vi "CRYOperator Process.vi"(9 "VI ID":i32=-1, 10 "sAction":string, 11 "sOperator Type":string) -> (3 "Data String":string)   [LabVIEW 2013]
uses:
  Control/CRYOperator Configure Cluster.ctl
  <vilib>/Utility/miscctls.llb/LVRectTypeDef.ctl
  SubVI/CRYMisc vis settings global.vi
panel:
  in  "Operator All Cluster":T1
  # "Register Operator Window."
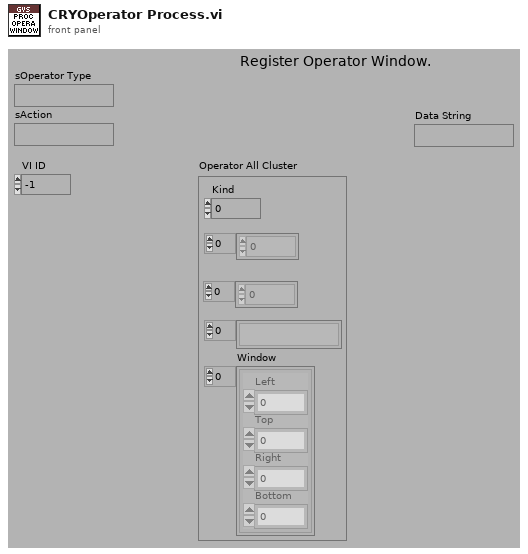
[diagram p1: front panel]
types:
  T1 = typedef "CRYOperator Configure Cluster.ctl" = cluster{"Kind":i32, "VI nID":i32[], "Title nID":i32[], "Setting":string[], "Window":T2[]}
  T2 = typedef "LVRectTypeDef.ctl" = cluster{"Left":i16, "Top":i16, "Right":i16, "Bottom":i16}
  T3 = cluster{"interactive":bool, "displayed":bool, "in a seq":bool}
  T4 = enum32{"Invalid", "Standard", "Closed", "Hidden", "Minimized", "Maximized"}
  T5 = enum32{"Invalid", "Default", "Floating", "Floating/Auto-Hide", "Modal"}
  T6 = cluster{"VI Ref":refnum<vi>[], "VI nID":i32[], "Title nID":i32[]}
  T7 = cluster{"gen'r mode":i32, "frequency":u32, "output level":dbl, "wave path":string, "wav play mode":i32, "duration":dbl, "n times":i32, "channel":i32, "wav level":dbl, "EQ":bool, "f knob log":bool, "f knob low":dbl, "f knob high":dbl, "ol knob log":bool, "ol knob low":dbl, "ol knob high":dbl, "Lin Display Prefs":string, "dB Display Prefs":string, "Duration noise":dbl, "Min freq noise":dbl, "Max freq noise":dbl, "Channel String":string, "Play Sine Wave":i32}
  T8 = typedef "CRYMultimeter.ctl" = cluster{"Ave/Max/Min":i32, "Level":i32, "Channel":i32, "Signal Type":string, "Weighting":string, "Applay Correction":bool, "lin/exp avg":u16, "rec time (sec)":dbl, "Average Time (Sec)":dbl, "Lin Display Prefs":string, "dB Display Prefs":string, "Time Weighting":u16, "Display":u16}
  T9 = typedef "CRYScope-FFT.ctl" = cluster{"window":i32, "n avgs":i32, "lin/exp avg":i32, "pwr/cplx avg":i32, "time (ms)":dbl, "fft lines":i32, "scope/fft mode":i32, "channel":i32, "trig. channel":i32, "Applay Correction":bool, "Time Display":string, "Freq. Weighting":string, "Ave/Max/Min":u16, "Trigger Level":dbl, "Trigger Unit":u16, "Trigger Time Offset":dbl, "Trigger Slope":u16, "Trigger/Free Run":bool, "continuous":bool, "Spectrum Display":string, "Calc FFT":bool, "Y-axis":string, "Signal Type":string}
  T10 = cluster{"octave":i32, "det time":i32, "det sec":dbl, "lin/exp":i32, "weighting":i32, "channel":i32, "Ave/Max/Min":u16, "continuous":bool, "Applay Correction":bool, "Display":u16, "Channel String":string}
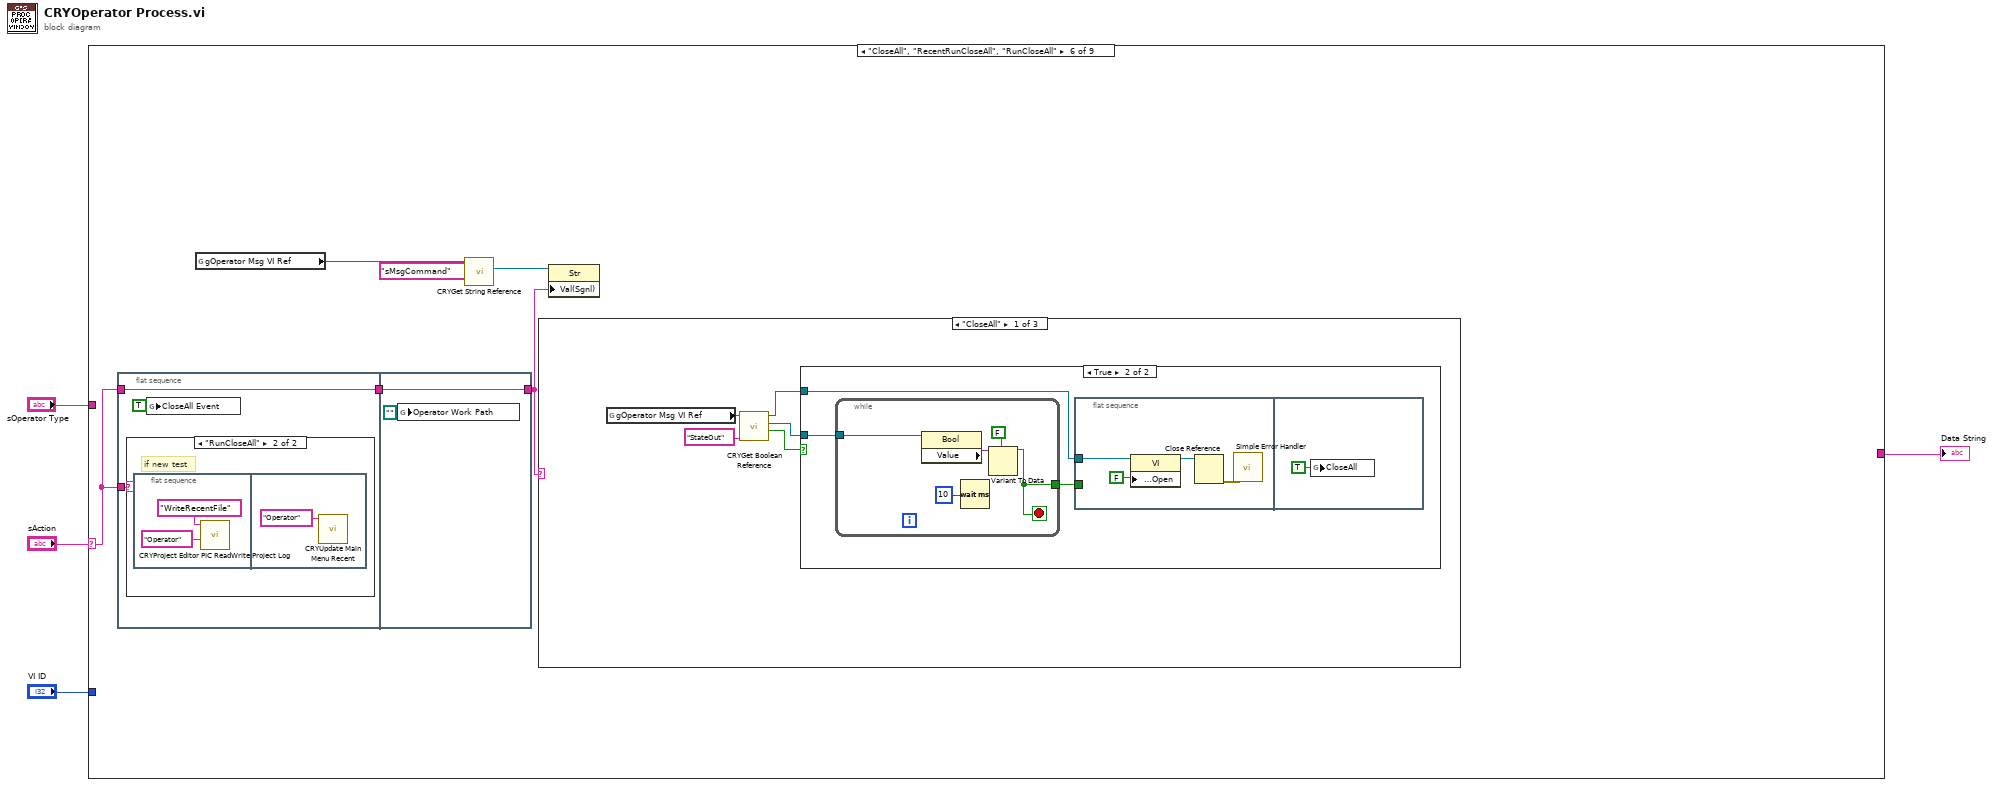
[diagram p0: block diagram]
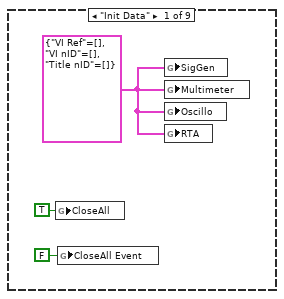
[diagram p2: hidden frame]
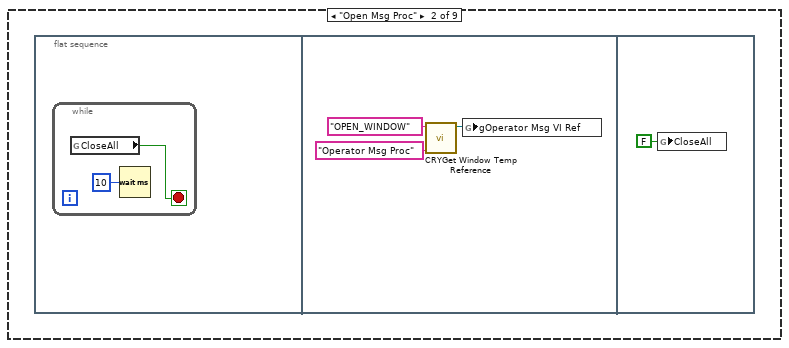
[diagram p3: hidden frame]
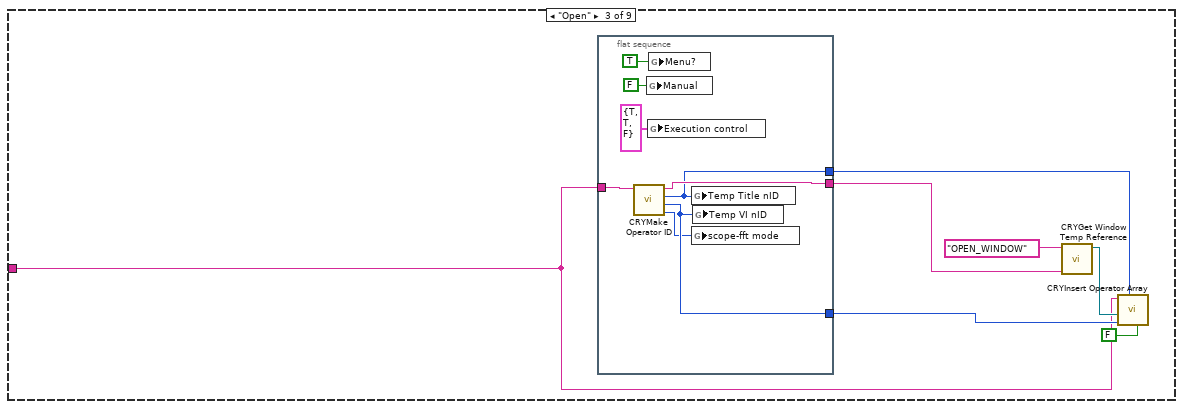
[diagram p4: hidden frame]
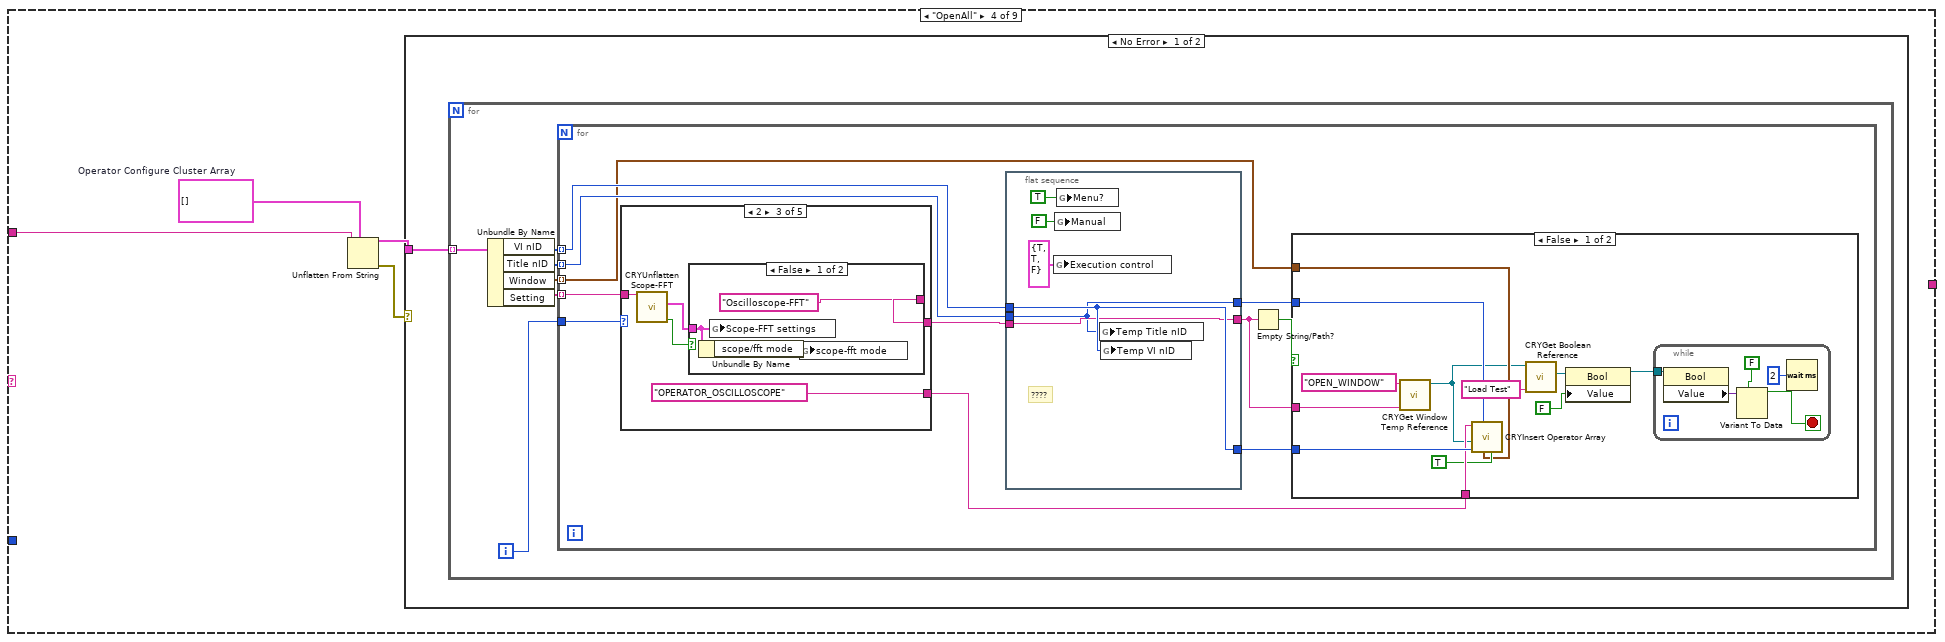
[diagram p5: hidden frame]
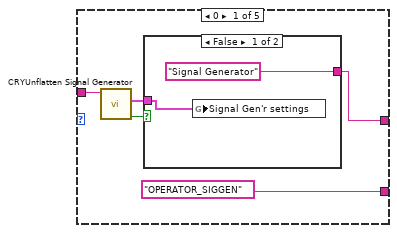
[diagram p7: hidden frame]
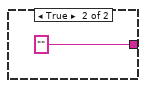
[diagram p8: hidden frame]
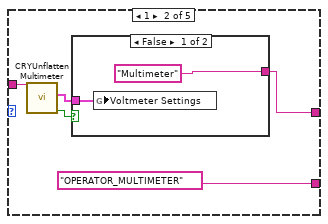
[diagram p9: hidden frame]
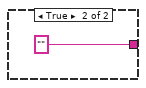
[diagram p10: hidden frame]
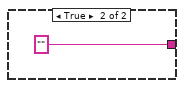
[diagram p11: hidden frame]
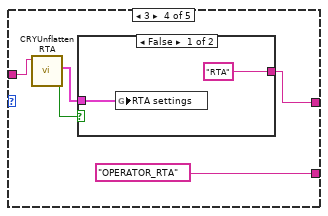
[diagram p12: hidden frame]
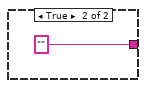
[diagram p13: hidden frame]
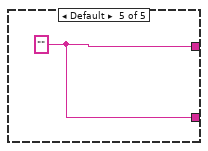
[diagram p14: hidden frame]
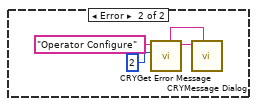
[diagram p15: hidden frame]
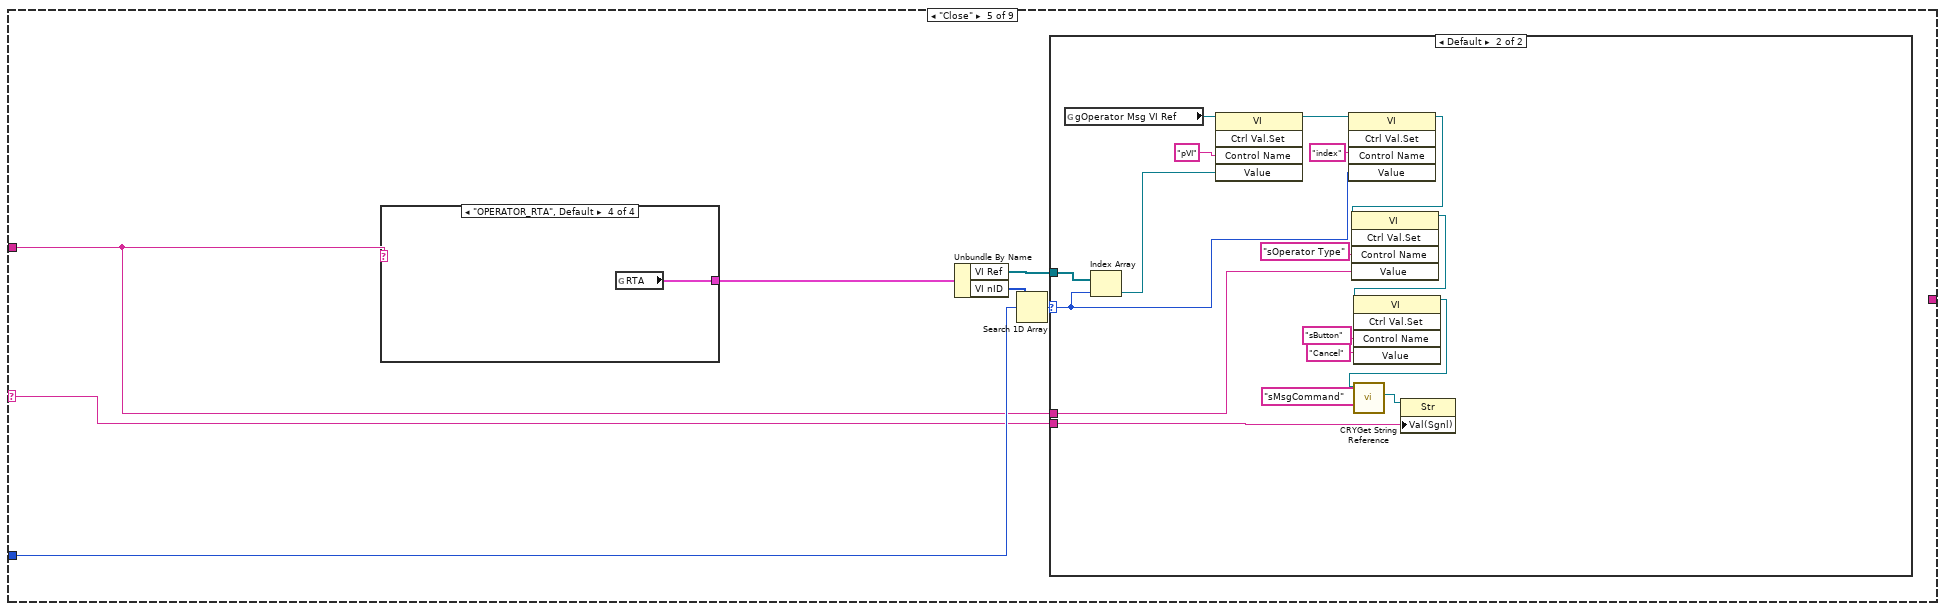
[diagram p16: hidden frame]
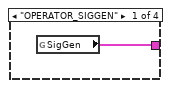
[diagram p18: hidden frame]
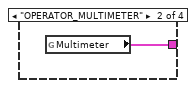
[diagram p19: hidden frame]
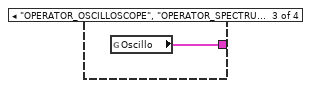
[diagram p20: hidden frame]
diagram:
  n1 = case shown="\"CloseAll\", \"RecentRunCloseAll\", \"RunCloseAll\"" "sAction" {
    selector: "sAction" -> [_ _ _ _ w112 w140 _ w326 _]
    tunnel: "sOperator Type" -> [_ _ w16 w31 w113 _ _ _ _]
    tunnel: "VI ID" -> [_ _ _ _ w117 _ _ _ _]
    tunnel: [_ _ _ _ _ _ w226 _ _] -> w1
    frame "Init Data" {
      w6 = T6 {"VI Ref"=[], "VI nID"=[], "Title nID"=[]} ("RTA")
      n2 = global write "CRYMisc vis settings global.vi" "CloseAll"(TRUE ("CloseAll")) -> ()
      n3 = global write "CRYMisc vis settings global.vi" "CloseAll Event"(FALSE ("CloseAll Event")) -> ()
      n4 = global write "CRYMisc vis settings global.vi" "SigGen"(w6) -> ()
      n5 = global write "CRYMisc vis settings global.vi" "Multimeter"(w6) -> ()
      n6 = global write "CRYMisc vis settings global.vi" "Oscillo"(w6) -> ()
      n7 = global write "CRYMisc vis settings global.vi" "RTA"(w6) -> ()
    }
    frame "Open Msg Proc" {
      n8 = flat-sequence {
        frame #0 {
          n9 = while {
            stop <- w8 stop-if-true
            n10 = global read "CRYMisc vis settings global.vi" "CloseAll"() -> (w8:bool)
            n11 = Wait (ms)(milliseconds to wait=u32 10) -> ()  [unwired: 1 out]
          }
        }
        frame #1 {
          n12 = call "CRYGet Window Temp Reference.vi"("sWindowName"="Operator Msg Proc", "sAction"="OPEN_WINDOW") -> ("pVIRef_Out"=w10:refnum<vi>)  [unwired: 5 in, 4 out]
          n13 = global write "CRYMisc vis settings global.vi" "gOperator Msg VI Ref"(w10) -> ()
        }
        frame #2 {
          n14 = global write "CRYMisc vis settings global.vi" "CloseAll"(FALSE ("CloseAll")) -> ()
        }
      }
    }
    frame "Open" {
      n15 = flat-sequence {
        tunnel: w16 -> [w25]
        tunnel: [w24] -> w18
        tunnel: [w23] -> w19
        tunnel: [w21] -> w14
        frame #0 {
          n16 = call "CRYMake Operator ID.vi"("sOperator Type"=w25) -> ("scope-fft mode"=w22:u32, "VI nID"=w23:i32, "Title ID"=w21:i32, "Window Name"=w24:string)  [unwired: 7 in]
          n17 = global write "CRYMisc vis settings global.vi" "Manual"(FALSE ("Mute")) -> ()
          n18 = global write "CRYMisc vis settings global.vi" "Execution control"(T3 {"interactive"=TRUE, "displayed"=TRUE, "in a seq"=FALSE} ("Execution control")) -> ()
          n19 = global write "CRYMisc vis settings global.vi" "Menu?"(TRUE ("Menu?")) -> ()
          n20 = global write "CRYMisc vis settings global.vi" "Temp Title nID"(w21) -> ()
          n21 = global write "CRYMisc vis settings global.vi" "scope-fft mode"(w22) -> ()
          n22 = global write "CRYMisc vis settings global.vi" "Temp VI nID"(w23) -> ()
        }
      }
      n23 = call "CRYGet Window Temp Reference.vi"("sWindowName"=w18, "sAction"="OPEN_WINDOW") -> ("pVIRef_Out"=w17:refnum<vi>)  [unwired: 5 in, 4 out]
      n24 = call "CRYInsert Operator Array.vi"("OpenAll/Open"=FALSE, "Title nID"=w14, "VI nID"=w19, "pVIRef_Out"=w17, "sOperator Type"=w16) -> ()  [unwired: 7 in]
    }
    frame "OpenAll" {
      w32 = T1[] []  # Operator Configure Cluster Array
      n25 = Unflatten From String(type=w32, binary string=w31) -> (value=w30:T1[], error out=w29:errorcluster)  [unwired: 3 in, 1 out]
      n26 = case shown="No Error" w29 {
        tunnel: w30 -> [w33 _]
        frame No Error {
          n27 = for {
            tunnel: w33 -> [w38] mode=indexing
            i -> [w39]
            n28 = Unbundle By Name(w38) -> ("VI nID"=w37:i32[], "Title nID"=w36:i32[], "Window"=w35:T2[], "Setting"=w34:string[])
            n29 = for {
              tunnel: w39 -> [w50]
              tunnel: w37 -> [w45] mode=indexing
              tunnel: w36 -> [w44] mode=indexing
              tunnel: w35 -> [w43] mode=indexing
              tunnel: w34 -> [w40] mode=indexing
              n30 = case shown="2" w50 {
                tunnel: ["OPERATOR_SIGGEN" ("sAction") "OPERATOR_MULTIMETER" ("sAction") "OPERATOR_OSCILLOSCOPE" ("sAction") "OPERATOR_RTA" ("sAction") w107] -> w48
                tunnel: [w75 w82 w90 w99 w107] -> w42
                tunnel: w40 -> [w77 w85 w93 w102 _]
                frame 0 {
                  n31 = call "CRYUnflatten Signal Generator.vi"("Flat Signal Gen'r settings"=w77) -> ("Error?"=w76:bool, "Signal Gen'r settings"=w74:T7)  [unwired: 8 in, 1 out]
                  n32 = case shown="False" w76 {
                    tunnel: ["Signal Generator" ("sAction") "" ("t")] -> w75
                    tunnel: w74 -> [w79 _]
                    frame False {
                      n33 = global write "CRYMisc vis settings global.vi" "Signal Gen'r settings"(w79) -> ()
                    }
                    frame True {
                    }
                  }
                }
                frame 1 {
                  n34 = call "CRYUnflatten Multimeter.vi"("Flat Voltmeter setup"=w85) -> ("Error?"=w83:bool, "Voltmeter Settings"=w84:T8)  [unwired: 8 in, 1 out]
                  n35 = case shown="False" w83 {
                    tunnel: ["Multimeter" ("sAction") "" ("t")] -> w82
                    tunnel: w84 -> [w88 _]
                    frame False {
                      n36 = global write "CRYMisc vis settings global.vi" "Voltmeter Settings"(w88) -> ()
                    }
                    frame True {
                    }
                  }
                }
                frame 2 {
                  n37 = call "CRYUnflatten Scope-FFT.vi"("Flat Scope-FFT setup"=w93) -> ("Error?"=w91:bool, "Scope-FFT settings"=w92:T9)  [unwired: 8 in, 1 out]
                  n38 = case shown="False" w91 {
                    tunnel: ["Oscilloscope-FFT" ("sAction") "" ("t")] -> w90
                    tunnel: w92 -> [w96 _]
                    frame False {
                      n39 = Unbundle By Name(w96) -> ("scope/fft mode"=w95:i32)
                      n40 = global write "CRYMisc vis settings global.vi" "Scope-FFT settings"(w96) -> ()
                      n41 = global write "CRYMisc vis settings global.vi" "scope-fft mode"(w95) -> ()
                    }
                    frame True {
                    }
                  }
                }
                frame 3 {
                  n42 = call "CRYUnflatten RTA.vi"("Flat RTA setup"=w102) -> ("Error?"=w100:bool, "RTA settings"=w101:T10)  [unwired: 8 in, 1 out]
                  n43 = case shown="False" w100 {
                    tunnel: ["RTA" ("sAction") "" ("t")] -> w99
                    tunnel: w101 -> [w105 _]
                    frame False {
                      n44 = global write "CRYMisc vis settings global.vi" "RTA settings"(w105) -> ()
                    }
                    frame True {
                    }
                  }
                }
                frame Default {
                  w107 = "" ("sAction")
                }
              }
              n45 = flat-sequence {
                tunnel: w42 -> [w69]
                tunnel: [w69] -> w47
                tunnel: [w70] -> w49
                tunnel: w45 -> [w70]
                tunnel: w44 -> [w68]
                tunnel: [w68] -> w41
                frame #0 {
                  # "????"
                  n46 = global write "CRYMisc vis settings global.vi" "Execution control"(T3 {"interactive"=TRUE, "displayed"=TRUE, "in a seq"=FALSE} ("Execution control")) -> ()
                  n47 = global write "CRYMisc vis settings global.vi" "Manual"(FALSE ("Mute")) -> ()
                  n48 = global write "CRYMisc vis settings global.vi" "Menu?"(TRUE ("Menu?")) -> ()
                  n49 = global write "CRYMisc vis settings global.vi" "Temp Title nID"(w68) -> ()
                  n50 = global write "CRYMisc vis settings global.vi" "Temp VI nID"(w70) -> ()
                }
              }
              n51 = Empty String/Path?(string/path=w47) -> (empty?=w46:bool)
              n52 = case shown="False" w46 {
                tunnel: w49 -> [w61 _]
                tunnel: w48 -> [w60 _]
                tunnel: w47 -> [w59 _]
                tunnel: w43 -> [w57 _]
                tunnel: w41 -> [w56 _]
                frame False {
                  n53 = call "CRYGet Window Temp Reference.vi"("sWindowName"=w59, "sAction"="OPEN_WINDOW") -> ("pVIRef_Out"=w55:refnum<vi>)  [unwired: 5 in, 4 out]
                  n54 = call "CRYInsert Operator Array.vi"("OpenAll/Open"=TRUE, "Front Panel Window:Window Bounds"=w57, "Title nID"=w56, "VI nID"=w61, "pVIRef_Out"=w55, "sOperator Type"=w60) -> ()  [unwired: 6 in]
                  n55 = call "CRYGet Boolean Reference.vi"("Label Name"="Load Test", "VI Refnum"=w55) -> ("Boolean Ref"=w53:refnum<vi>)  [unwired: 7 in, 2 out]
                  n56 = property class="Bool"(reference=w53, "Value"=FALSE ("OpenAll/Open")) -> (reference out=w51:refnum<vi>)  [unwired: 1 in, 1 out]
                  n57 = while {
                    tunnel: w51 -> [w67]
                    stop <- w64 stop-if-true
                    n58 = property class="Bool"(reference=w67) -> ("Value"=w65:variant)  [unwired: 1 in, 2 out]
                    n59 = Variant To Data(type=FALSE ("OpenAll/Open"), Variant=w65) -> (data=w64:bool)  [unwired: 1 in, 1 out]
                    n60 = Wait (ms)(milliseconds to wait=u32 2) -> ()  [unwired: 1 out]
                  }
                }
                frame True {
                }
              }
            }
          }
        }
        frame Error {
          n61 = call "CRYGet Error Message.vi"("Error No"=2, "Kind"="Operator Configure") -> ("Message"=w111:string, "Window Title"=w110:string)  [unwired: 4 in, 4 out]
          n62 = call "CRYMessage Dialog.vi"("Window Title"=w110, "Message Content"=w111) -> ()  [unwired: 8 in, 2 out]
        }
      }
    }
    frame "Close" {
      n63 = case shown="\"OPERATOR_RTA\", Default" w113 {
        tunnel: [w136 w137 w138 w139] -> w114
        frame "OPERATOR_SIGGEN" {
          n64 = global read "CRYMisc vis settings global.vi" "SigGen"() -> (w136:T6)
        }
        frame "OPERATOR_MULTIMETER" {
          n65 = global read "CRYMisc vis settings global.vi" "Multimeter"() -> (w137:T6)
        }
        frame "OPERATOR_OSCILLOSCOPE", "OPERATOR_SPECTRUM" {
          n66 = global read "CRYMisc vis settings global.vi" "Oscillo"() -> (w138:T6)
        }
        frame "OPERATOR_RTA", Default {
          n67 = global read "CRYMisc vis settings global.vi" "RTA"() -> (w139:T6)
        }
      }
      n68 = Unbundle By Name(w114) -> ("VI Ref"=w115:refnum<vi>[], "VI nID"=w118:i32[])
      n69 = Search 1D Array(1D array=w118, element=w117) -> (index of element=w116:i32)  [unwired: 1 in]
      n70 = case shown="Default" w116 {
        selector: w116 -> [_ w125]
        tunnel: w115 -> [_ w135]
        tunnel: w113 -> [_ w124]
        tunnel: w112 -> [_ w120]
        frame -1 {
        }
        frame Default {
          n71 = global read "CRYMisc vis settings global.vi" "gOperator Msg VI Ref"() -> (w130:refnum<vi>)
          n72 = Index Array(array=w135, index=w125) -> (element=w133:refnum<vi>)
          n73 = invoke class="VI" method="Ctrl Val.Set"(reference=w130, "Control Name"="pVI", "Value"=w133) -> (reference out=w129:refnum<vi>)  [unwired: 2 in, 4 out]
          n74 = invoke class="VI" method="Ctrl Val.Set"(reference=w129, "Control Name"="index", "Value"=w125) -> (reference out=w128:refnum<vi>)  [unwired: 2 in, 4 out]
          n75 = invoke class="VI" method="Ctrl Val.Set"(reference=w128, "Control Name"="sOperator Type", "Value"=w124) -> (reference out=w122:refnum<vi>)  [unwired: 2 in, 4 out]
          n76 = invoke class="VI" method="Ctrl Val.Set"(reference=w122, "Control Name"="sButton", "Value"="Cancel" ("Label Name")) -> (reference out=w121:refnum<vi>)  [unwired: 2 in, 4 out]
          n77 = call "CRYGet String Reference.vi"("Label Name"="sMsgCommand" ("Control Name"), "VI Refnum"=w121) -> ("String Ref Out"=w131:refnum<vi>)  [unwired: 7 in, 2 out]
          n78 = property class="Str"(reference=w131, "Val(Sgnl)"=w120) -> ()  [unwired: 1 in, 2 out]
        }
      }
    }
    frame "CloseAll", "RecentRunCloseAll", "RunCloseAll" {
      n79 = flat-sequence {
        tunnel: w140 -> [w147]
        tunnel: [w147] -> w141
        tunnel: w140 -> [w146]
        tunnel: [w153] -> w142
        tunnel: w141 -> [w153]
        frame #0 {
          n80 = case shown="\"RunCloseAll\"" w146 {
            frame "False", Default {
            }
            frame "RunCloseAll" {
              # "if new test"
              n81 = flat-sequence {
                frame #0 {
                  n82 = call "CRYProject Editor PIC ReadWrite Project Log.vi"("sData"="Operator", "sAction"="WriteRecentFile") -> ()  [unwired: 8 in, 2 out]
                }
                frame #1 {
                  n83 = call "CRYUpdate Main Menu Recent.vi"("menu tag"="Operator") -> ()  [unwired: 11 in]
                }
              }
            }
          }
          n84 = global write "CRYMisc vis settings global.vi" "CloseAll Event"(TRUE ("CloseAll Event")) -> ()
        }
        frame #1 {
          n85 = global write "CRYMisc vis settings global.vi" "Operator Work Path"(path "") -> ()
        }
      }
      n86 = global read "CRYMisc vis settings global.vi" "gOperator Msg VI Ref"() -> (w143:refnum<vi>)
      n87 = call "CRYGet String Reference.vi"("Label Name"="sMsgCommand" ("Control Name"), "VI Refnum"=w143) -> ("String Ref Out"=w145:refnum<vi>)  [unwired: 7 in, 2 out]
      n88 = case shown="\"CloseAll\"" w142 {
        frame "CloseAll" {
          n89 = global read "CRYMisc vis settings global.vi" "gOperator Msg VI Ref"() -> (w158:refnum<vi>)
          n90 = call "CRYGet Boolean Reference.vi"("Label Name"="StateOut", "VI Refnum"=w158) -> ("Exist?"=w154:bool, "Boolean Ref"=w155:refnum<vi>, "VI Refnum Out"=w156:refnum<vi>)  [unwired: 7 in]
          n91 = case shown="True" w154 {
            tunnel: w155 -> [_ w161]
            tunnel: w156 -> [_ w159]
            frame False {
            }
            frame True {
              n92 = while {
                tunnel: w161 -> [w171]
                tunnel: [w168] -> w160
                stop <- w168 stop-if-true
                n93 = property class="Bool"(reference=w171) -> ("Value"=w170:variant)  [unwired: 1 in, 2 out]
                n94 = Wait (ms)(milliseconds to wait=u32 10) -> ()  [unwired: 1 out]
                n95 = Variant To Data(type=FALSE ("Boolean"), Variant=w170) -> (data=w168:bool)  [unwired: 1 in, 1 out]
              }
              n96 = flat-sequence {
                tunnel: w159 -> [w165]
                tunnel: w160 -> [_]
                frame #0 {
                  n97 = property class="VI"(reference=w165, "Front Panel.Open"=FALSE ("Front Panel Window:Open")) -> (reference out=w164:refnum<vi>)  [unwired: 1 in, 1 out]
                  n98 = Close Reference(reference=w164) -> (error out=w162:errorcluster)  [unwired: 1 in]
                  n99 = call <vilib>:"Simple Error Handler.vi"("error in (no error)"=w162) -> ()  [unwired: 2 in, 7 out]
                }
                frame #1 {
                  n100 = global write "CRYMisc vis settings global.vi" "CloseAll"(TRUE ("CloseAll")) -> ()
                }
              }
            }
          }
        }
        frame "RecentRunCloseAll", "RunCloseAll" {
          n101 = flat-sequence {
            tunnel: [w173] -> w172
            frame #0 {
              n102 = while {
                tunnel: [w174] -> w173
                stop <- w174 stop-if-true
                n103 = global read "CRYMisc vis settings global.vi" "CloseAll Event"() -> (w176:bool)
                n104 = Wait (ms)(milliseconds to wait=u32 2) -> ()  [unwired: 1 out]
                n105 = Not(x=w176) -> (.not. x?=w174:bool)
              }
            }
          }
          n106 = while {
            tunnel: w172 -> [_]
            stop <- w178 stop-if-true
            n107 = global read "CRYMisc vis settings global.vi" "Multimeter"() -> (w180:T6)
            n108 = global read "CRYMisc vis settings global.vi" "SigGen"() -> (w179:T6)
            n109 = global read "CRYMisc vis settings global.vi" "Oscillo"() -> (w181:T6)
            n110 = global read "CRYMisc vis settings global.vi" "RTA"() -> (w182:T6)
            n111 = Unbundle By Name(w179) -> ("VI Ref"=w183:refnum<vi>[])
            n112 = Unbundle By Name(w180) -> ("VI Ref"=w184:refnum<vi>[])
            n113 = Unbundle By Name(w181) -> ("VI Ref"=w185:refnum<vi>[])
            n114 = Unbundle By Name(w182) -> ("VI Ref"=w186:refnum<vi>[])
            n115 = Array Size(array=w183) -> (size(s)=w187:i32)
            n116 = Array Size(array=w184) -> (size(s)=w188:i32)
            n117 = Array Size(array=w185) -> (size(s)=w189:i32)
            n118 = Array Size(array=w186) -> (size(s)=w190:i32)
            n119 = Equal To 0?(x=w187) -> (x = 0?=w191:bool)
            n120 = Equal To 0?(x=w188) -> (x = 0?=w192:bool)
            n121 = Equal To 0?(x=w189) -> (x = 0?=w193:bool)
            n122 = Equal To 0?(x=w190) -> (x = 0?=w194:bool)
            n123 = Compound Arithmetic op=AND(w191, w192, w193, w194) -> (w178:bool)
            n124 = Wait (ms)(milliseconds to wait=u32 2) -> ()  [unwired: 1 out]
          }
        }
        frame Default {
        }
      }
      n125 = property class="Str"(reference=w145, "Val(Sgnl)"=w142) -> ()  [unwired: 1 in, 2 out]
    }
    frame "GetStateAll" {
      n126 = global read "CRYMisc vis settings global.vi" "Multimeter"() -> (w229:T6)
      n127 = global read "CRYMisc vis settings global.vi" "SigGen"() -> (w237:T6)
      n128 = global read "CRYMisc vis settings global.vi" "Oscillo"() -> (w227:T6)
      n129 = global read "CRYMisc vis settings global.vi" "RTA"() -> (w228:T6)
      n130 = Unbundle By Name(w237) -> ("VI Ref"=w236:refnum<vi>[], "VI nID"=w235:i32[], "Title nID"=w196:i32[])
      n131 = Unbundle By Name(w229) -> ("VI Ref"=w220:refnum<vi>[], "VI nID"=w219:i32[], "Title nID"=w200:i32[])
      n132 = Unbundle By Name(w227) -> ("VI Ref"=w222:refnum<vi>[], "VI nID"=w221:i32[], "Title nID"=w204:i32[])
      n133 = Unbundle By Name(w228) -> ("VI Ref"=w224:refnum<vi>[], "VI nID"=w223:i32[], "Title nID"=w208:i32[])
      n134 = for {
        tunnel: w222 -> [w264] mode=indexing
        tunnel: w221 -> [w272] mode=indexing
        tunnel: [w272] -> w217 mode=indexing
        tunnel: [w259] -> w205 mode=indexing
        tunnel: [w271] -> w206 mode=indexing
        tunnel: [w262] -> w203 mode=indexing
        tunnel: w204 -> [w262] mode=indexing
        n135 = call "CRYGet Boolean Reference.vi"("Label Name"="Set Configure" ("Control Name"), "VI Refnum"=w264) -> ("Boolean Ref"=w268:refnum<vi>)  [unwired: 7 in, 2 out]
        n136 = property class="Bool"(reference=w268, "Val(Sgnl)"=FALSE) -> (reference out=w267:refnum<vi>)  [unwired: 1 in, 1 out]
        n137 = while {
          tunnel: w267 -> [w278]
          tunnel: [w274] -> w265
          tunnel: w264 -> [w274]
          stop <- w275 stop-if-true
          n138 = property class="Bool"(reference=w278) -> ("Value"=w276:variant)  [unwired: 1 in, 2 out]
          n139 = Wait (ms)(milliseconds to wait=u32 2) -> ()  [unwired: 1 out]
          n140 = Variant To Data(type=FALSE, Variant=w276) -> (data=w275:bool)  [unwired: 1 in, 1 out]
        }
        n141 = invoke class="VI" method="Ctrl Val.Get"(reference=w265, "Control Name"="Configure Data") -> (reference out=w263:refnum<vi>, error out=w270:errorcluster, "Get Control Value Variant"=w261:variant)  [unwired: 2 in, 1 out]
        n142 = property class="VI"(reference=w263, error in=w270) -> ("Front Panel.WinBounds"=w271:T2)  [unwired: 2 out]
        n143 = Variant To Data(type="" ("Data Name"), Variant=w261) -> (data=w259:string)  [unwired: 1 in, 1 out]
      }
      n144 = for {
        tunnel: w236 -> [w306] mode=indexing
        tunnel: w235 -> [w314] mode=indexing
        tunnel: [w314] -> w234 mode=indexing
        tunnel: [w301] -> w197 mode=indexing
        tunnel: [w313] -> w198 mode=indexing
        tunnel: w196 -> [w304] mode=indexing
        tunnel: [w304] -> w195 mode=indexing
        n145 = call "CRYGet Boolean Reference.vi"("Label Name"="Set Configure" ("Control Name"), "VI Refnum"=w306) -> ("Boolean Ref"=w310:refnum<vi>)  [unwired: 7 in, 2 out]
        n146 = property class="Bool"(reference=w310, "Val(Sgnl)"=FALSE) -> (reference out=w309:refnum<vi>)  [unwired: 1 in, 1 out]
        n147 = while {
          tunnel: w309 -> [w320]
          tunnel: [w316] -> w307
          tunnel: w306 -> [w316]
          stop <- w317 stop-if-true
          n148 = property class="Bool"(reference=w320) -> ("Value"=w318:variant)  [unwired: 1 in, 2 out]
          n149 = Wait (ms)(milliseconds to wait=u32 2) -> ()  [unwired: 1 out]
          n150 = Variant To Data(type=FALSE, Variant=w318) -> (data=w317:bool)  [unwired: 1 in, 1 out]
        }
        n151 = invoke class="VI" method="Ctrl Val.Get"(reference=w307, "Control Name"="Configure Data") -> (reference out=w305:refnum<vi>, error out=w312:errorcluster, "Get Control Value Variant"=w302:variant)  [unwired: 2 in, 1 out]
        n152 = property class="VI"(reference=w305, error in=w312) -> ("Front Panel.WinBounds"=w313:T2)  [unwired: 2 out]
        n153 = Variant To Data(type="" ("Data Name"), Variant=w302) -> (data=w301:string)  [unwired: 1 in, 1 out]
      }
      n154 = for {
        tunnel: w220 -> [w285] mode=indexing
        tunnel: w219 -> [w293] mode=indexing
        tunnel: [w293] -> w218 mode=indexing
        tunnel: [w280] -> w201 mode=indexing
        tunnel: [w292] -> w202 mode=indexing
        tunnel: w200 -> [w283] mode=indexing
        tunnel: [w283] -> w199 mode=indexing
        n155 = call "CRYGet Boolean Reference.vi"("Label Name"="Set Configure" ("Control Name"), "VI Refnum"=w285) -> ("Boolean Ref"=w289:refnum<vi>)  [unwired: 7 in, 2 out]
        n156 = property class="Bool"(reference=w289, "Val(Sgnl)"=FALSE) -> (reference out=w288:refnum<vi>)  [unwired: 1 in, 1 out]
        n157 = while {
          tunnel: w288 -> [w299]
          tunnel: [w295] -> w286
          tunnel: w285 -> [w295]
          stop <- w296 stop-if-true
          n158 = property class="Bool"(reference=w299) -> ("Value"=w297:variant)  [unwired: 1 in, 2 out]
          n159 = Wait (ms)(milliseconds to wait=u32 2) -> ()  [unwired: 1 out]
          n160 = Variant To Data(type=FALSE, Variant=w297) -> (data=w296:bool)  [unwired: 1 in, 1 out]
        }
        n161 = invoke class="VI" method="Ctrl Val.Get"(reference=w286, "Control Name"="Configure Data") -> (reference out=w284:refnum<vi>, error out=w291:errorcluster, "Get Control Value Variant"=w281:variant)  [unwired: 2 in, 1 out]
        n162 = property class="VI"(reference=w284, error in=w291) -> ("Front Panel.WinBounds"=w292:T2)  [unwired: 2 out]
        n163 = Variant To Data(type="" ("Data Name"), Variant=w281) -> (data=w280:string)  [unwired: 1 in, 1 out]
      }
      n164 = for {
        tunnel: w224 -> [w243] mode=indexing
        tunnel: w223 -> [w251] mode=indexing
        tunnel: [w251] -> w216 mode=indexing
        tunnel: [w238] -> w209 mode=indexing
        tunnel: [w250] -> w210 mode=indexing
        tunnel: w208 -> [w241] mode=indexing
        tunnel: [w241] -> w207 mode=indexing
        n165 = call "CRYGet Boolean Reference.vi"("Label Name"="Set Configure" ("Control Name"), "VI Refnum"=w243) -> ("Boolean Ref"=w247:refnum<vi>)  [unwired: 7 in, 2 out]
        n166 = property class="Bool"(reference=w247, "Val(Sgnl)"=FALSE) -> (reference out=w246:refnum<vi>)  [unwired: 1 in, 1 out]
        n167 = while {
          tunnel: w246 -> [w257]
          tunnel: [w253] -> w244
          tunnel: w243 -> [w253]
          stop <- w254 stop-if-true
          n168 = property class="Bool"(reference=w257) -> ("Value"=w255:variant)  [unwired: 1 in, 2 out]
          n169 = Wait (ms)(milliseconds to wait=u32 2) -> ()  [unwired: 1 out]
          n170 = Variant To Data(type=FALSE, Variant=w255) -> (data=w254:bool)  [unwired: 1 in, 1 out]
        }
        n171 = invoke class="VI" method="Ctrl Val.Get"(reference=w244, "Control Name"="Configure Data") -> (reference out=w242:refnum<vi>, error out=w249:errorcluster, "Get Control Value Variant"=w239:variant)  [unwired: 2 in, 1 out]
        n172 = property class="VI"(reference=w242, error in=w249) -> ("Front Panel.WinBounds"=w250:T2)  [unwired: 2 out]
        n173 = Variant To Data(type="" ("Data Name"), Variant=w239) -> (data=w238:string)  [unwired: 1 in, 1 out]
      }
      n174 = Bundle(cluster="Operator All Cluster", "Kind"=1, "VI nID"=w234, "Title nID"=w195, "Setting"=w197, "Window"=w198) -> (w215:T1)
      n175 = Bundle(cluster="Operator All Cluster", "Kind"=2, "VI nID"=w218, "Title nID"=w199, "Setting"=w201, "Window"=w202) -> (w214:T1)
      n176 = Bundle(cluster="Operator All Cluster", "Kind"=4, "VI nID"=w216, "Title nID"=w207, "Setting"=w209, "Window"=w210) -> (w212:T1)
      n177 = Bundle(cluster="Operator All Cluster", "Kind"=3, "VI nID"=w217, "Title nID"=w203, "Setting"=w205, "Window"=w206) -> (w213:T1)
      n178 = Build Array(w215, w214, w213, w212) -> (w211:T1[])
      n179 = Flatten To String(anything=w211) -> (data string=w226:string)  [unwired: 3 in, 2 out]
    }
    frame "Maximize", "Minimize" {
      n180 = Equal?(x=w326, y="Maximize" ("sAction")) -> (x = y?=w330:bool)
      n181 = Equal?(x=w326, y="Minimize" ("sAction")) -> (x = y?=w325:bool)
      n182 = Select(t=T4."Minimized" ("Front Panel Window:State"), s=w325, f=T4."Standard" ("Front Panel Window:State")) -> (s? t:f=w322:T4)
      n183 = global read "CRYMisc vis settings global.vi" "Multimeter"() -> (w333:T6)
      n184 = Select(t=T4."Standard" ("Front Panel Window:State"), s=w330, f=w322) -> (s? t:f=w328:T4)
      n185 = global read "CRYMisc vis settings global.vi" "SigGen"() -> (w332:T6)
      n186 = global read "CRYMisc vis settings global.vi" "Oscillo"() -> (w334:T6)
      n187 = global read "CRYMisc vis settings global.vi" "RTA"() -> (w335:T6)
      n188 = Unbundle By Name(w332) -> ("VI Ref"=w336:refnum<vi>[])
      n189 = Unbundle By Name(w333) -> ("VI Ref"=w337:refnum<vi>[])
      n190 = Unbundle By Name(w334) -> ("VI Ref"=w338:refnum<vi>[])
      n191 = Unbundle By Name(w335) -> ("VI Ref"=w339:refnum<vi>[])
      n192 = Build Array (concatenate)(w336, w337, w338, w339) -> (w340:refnum<vi>[])
      n193 = for {
        tunnel: w340 -> [w343] mode=indexing
        tunnel: w328 -> [w342]
        n194 = property class="VI"(reference=w343, "FP.State"=w342, "FP.Behavior"=T5."Floating" ("Front Panel Window:Behavior")) -> ()  [unwired: 1 in, 2 out]
      }
    }
    frame Default {
    }
  }
  "Data String" <- w1
